vi "main.vi"() -> ()   [LabVIEW 2016]
uses:
  <vilib>/DAQmx/read.llb/DAQmx Read (Analog 2D DBL NChan NSamp).vi
  <vilib>/DAQmx/miscellaneous.llb/DAQmx Fill In Error Info.vi
  QSM-PC (String)/Library/QSM-PC (String).lvlib
  <resource>/objmgr/daqmx.rc
panel:
  out "error out 3":errorcluster caption="错误输出"
  out "控件值:获取全部 2":cluster{"Name":string, "Variant Data":variant}[](array[cluster])
  out "输出簇":T1
  in  "Function":bool
  in  "Oscilloscope":bool
  out "DevName":string
  out "DCVoltage":dbl
  out "ai taskhandle":refnum<k21>
  out "error out read ai":errorcluster caption="error out"
  out "taskArr out create task out":refnum<k21>[](array[refnum])
  out "taskArr out create task in":refnum<k21>[](array[refnum])
  out "isDeviceExist":bool
  out "isNull":bool
  out "taskArr out":refnum<k21>[](array[refnum])
  out "error out 2":errorcluster caption="error out"
  out "error out":errorcluster
  out "msg from wrapper":cluster{"State":string, "Data":variant}
  in  "Creat_Task":bool
  out "AI":dbl[][](array[numeric])
  in  "Search_Drive":bool
  out "控件值:获取全部":cluster{"Name":string, "Variant Data":variant}[](array[cluster])
  out "QSM - Main":refnum<queue>
  out "R":dbl
  in  "调零测量":bool
  in  "start AI":bool
  in  "Stop":bool
  in  "Read R":bool
  in  "event registration refnum":refnum<event-registration>
  in  "user event out":refnum<user-event>
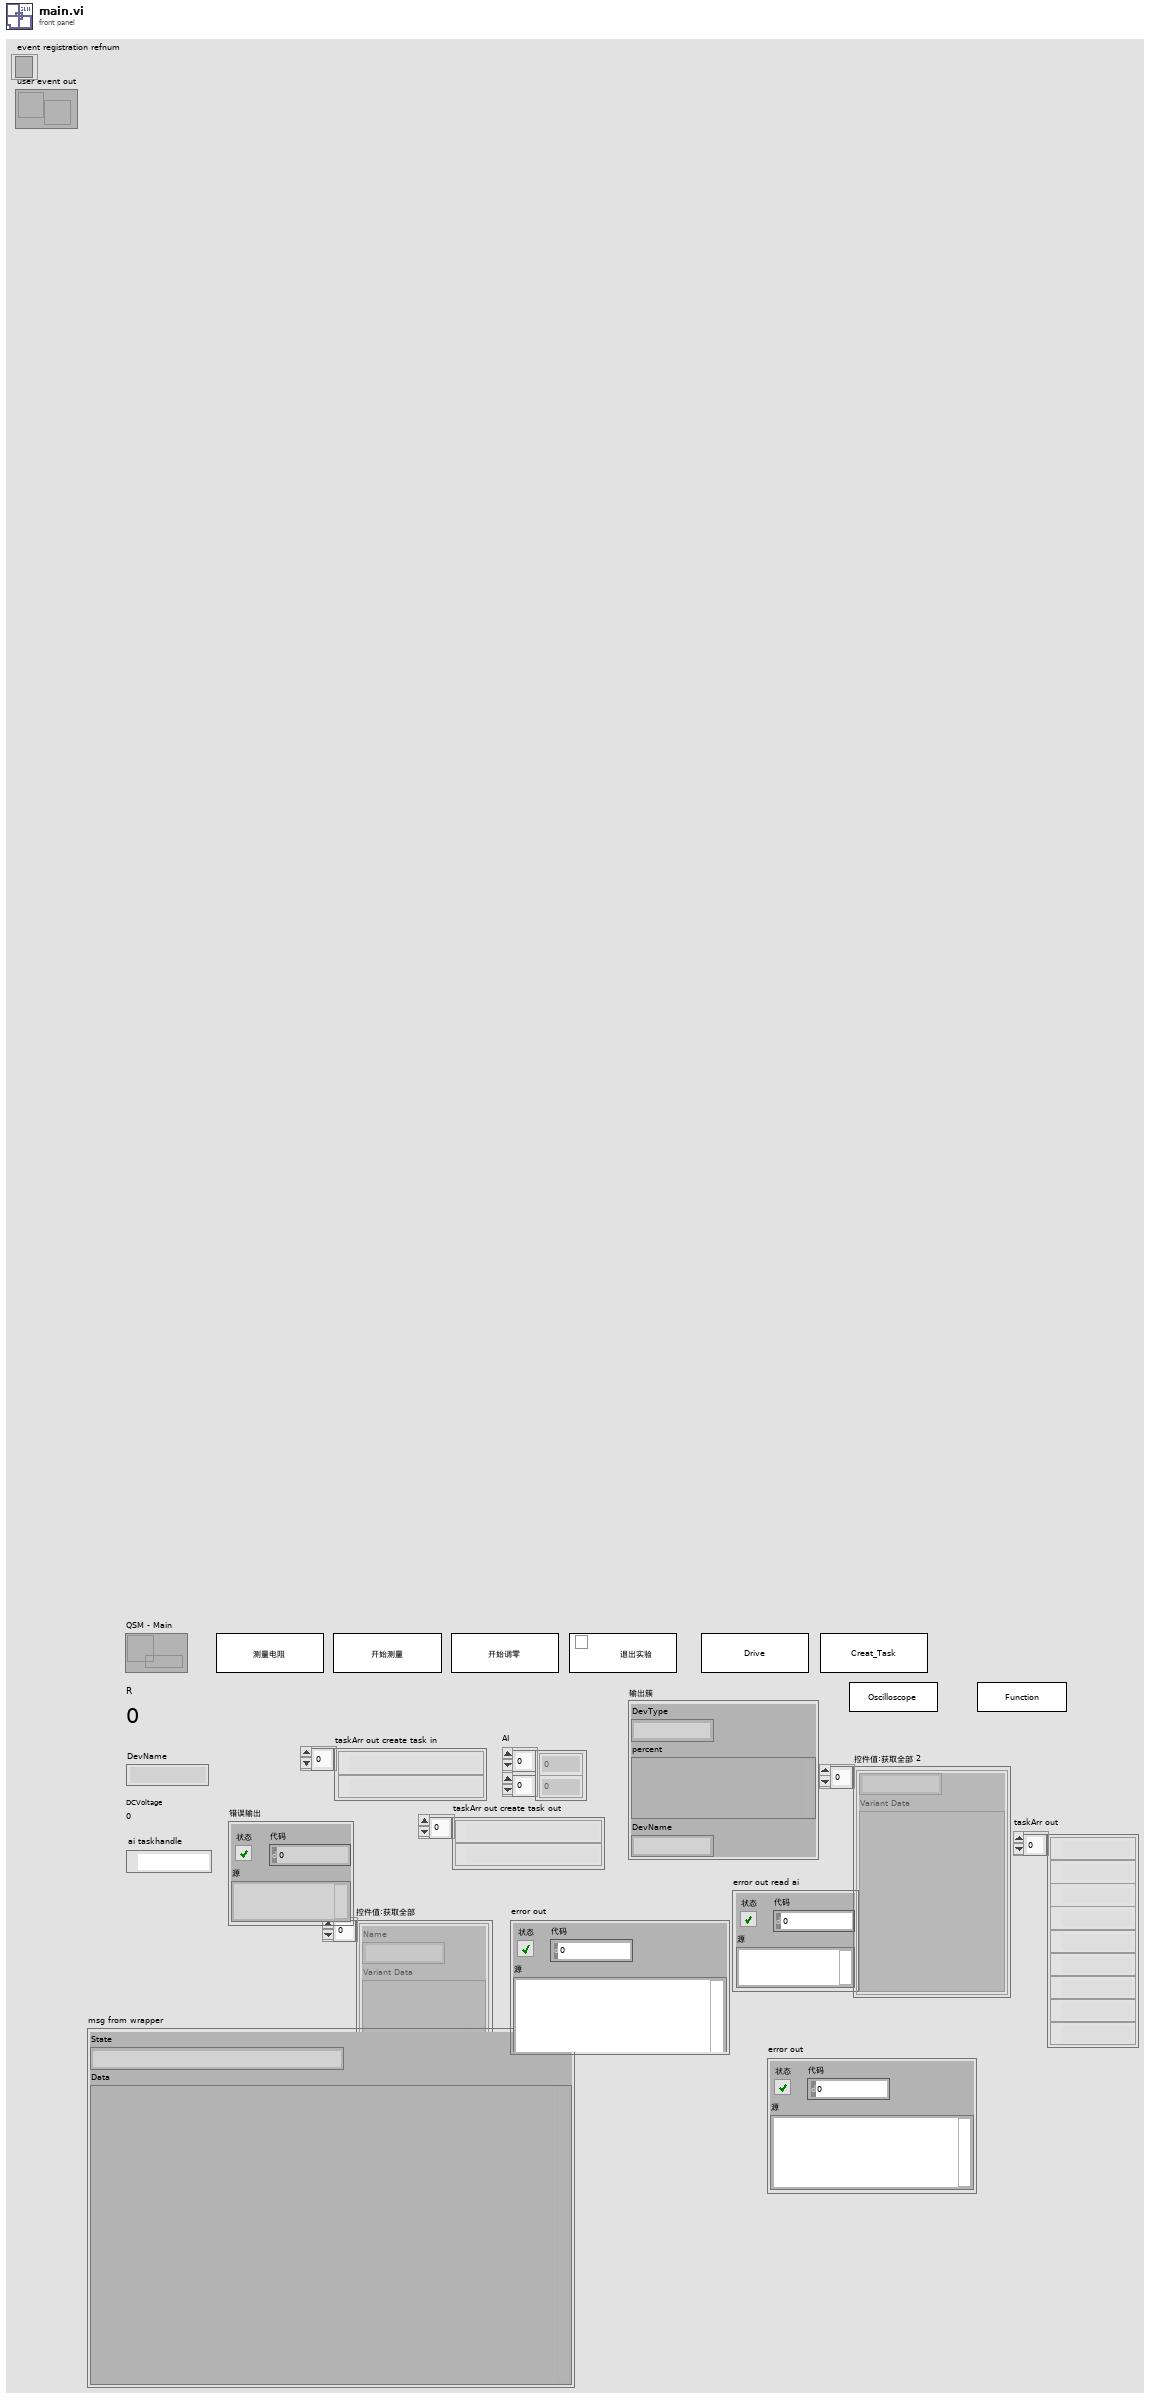
[diagram p1: front panel]
types:
  T1 = cluster{"DevType":string, "percent":variant, "DevName":string}
  T2 = cluster{"Oscilloscope":refnum<queue>, "Function":refnum<queue>}
  T3 = cluster{"DevType":string, "percent":dbl, "DevName":string}
  T4 = cluster{"DevType":string, "DevName":string, "Function":variant}
  T5 = typedef "Configuration.ctl" = cluster{"tasks":T6[]}
  T6 = typedef "TaskConfig.ctl" = cluster{"type":string, "channels":T7[], "sampleclock":T8}
  T7 = typedef "ChanConfig.ctl" = cluster{"physicalchanname":string, "max":dbl, "min":dbl}
  T8 = typedef "ClockConfig.ctl" = cluster{"rate":dbl, "samplesperchannel":i32}
  T9 = cluster{"Config":T5, "DevName":string, "DevType":string}
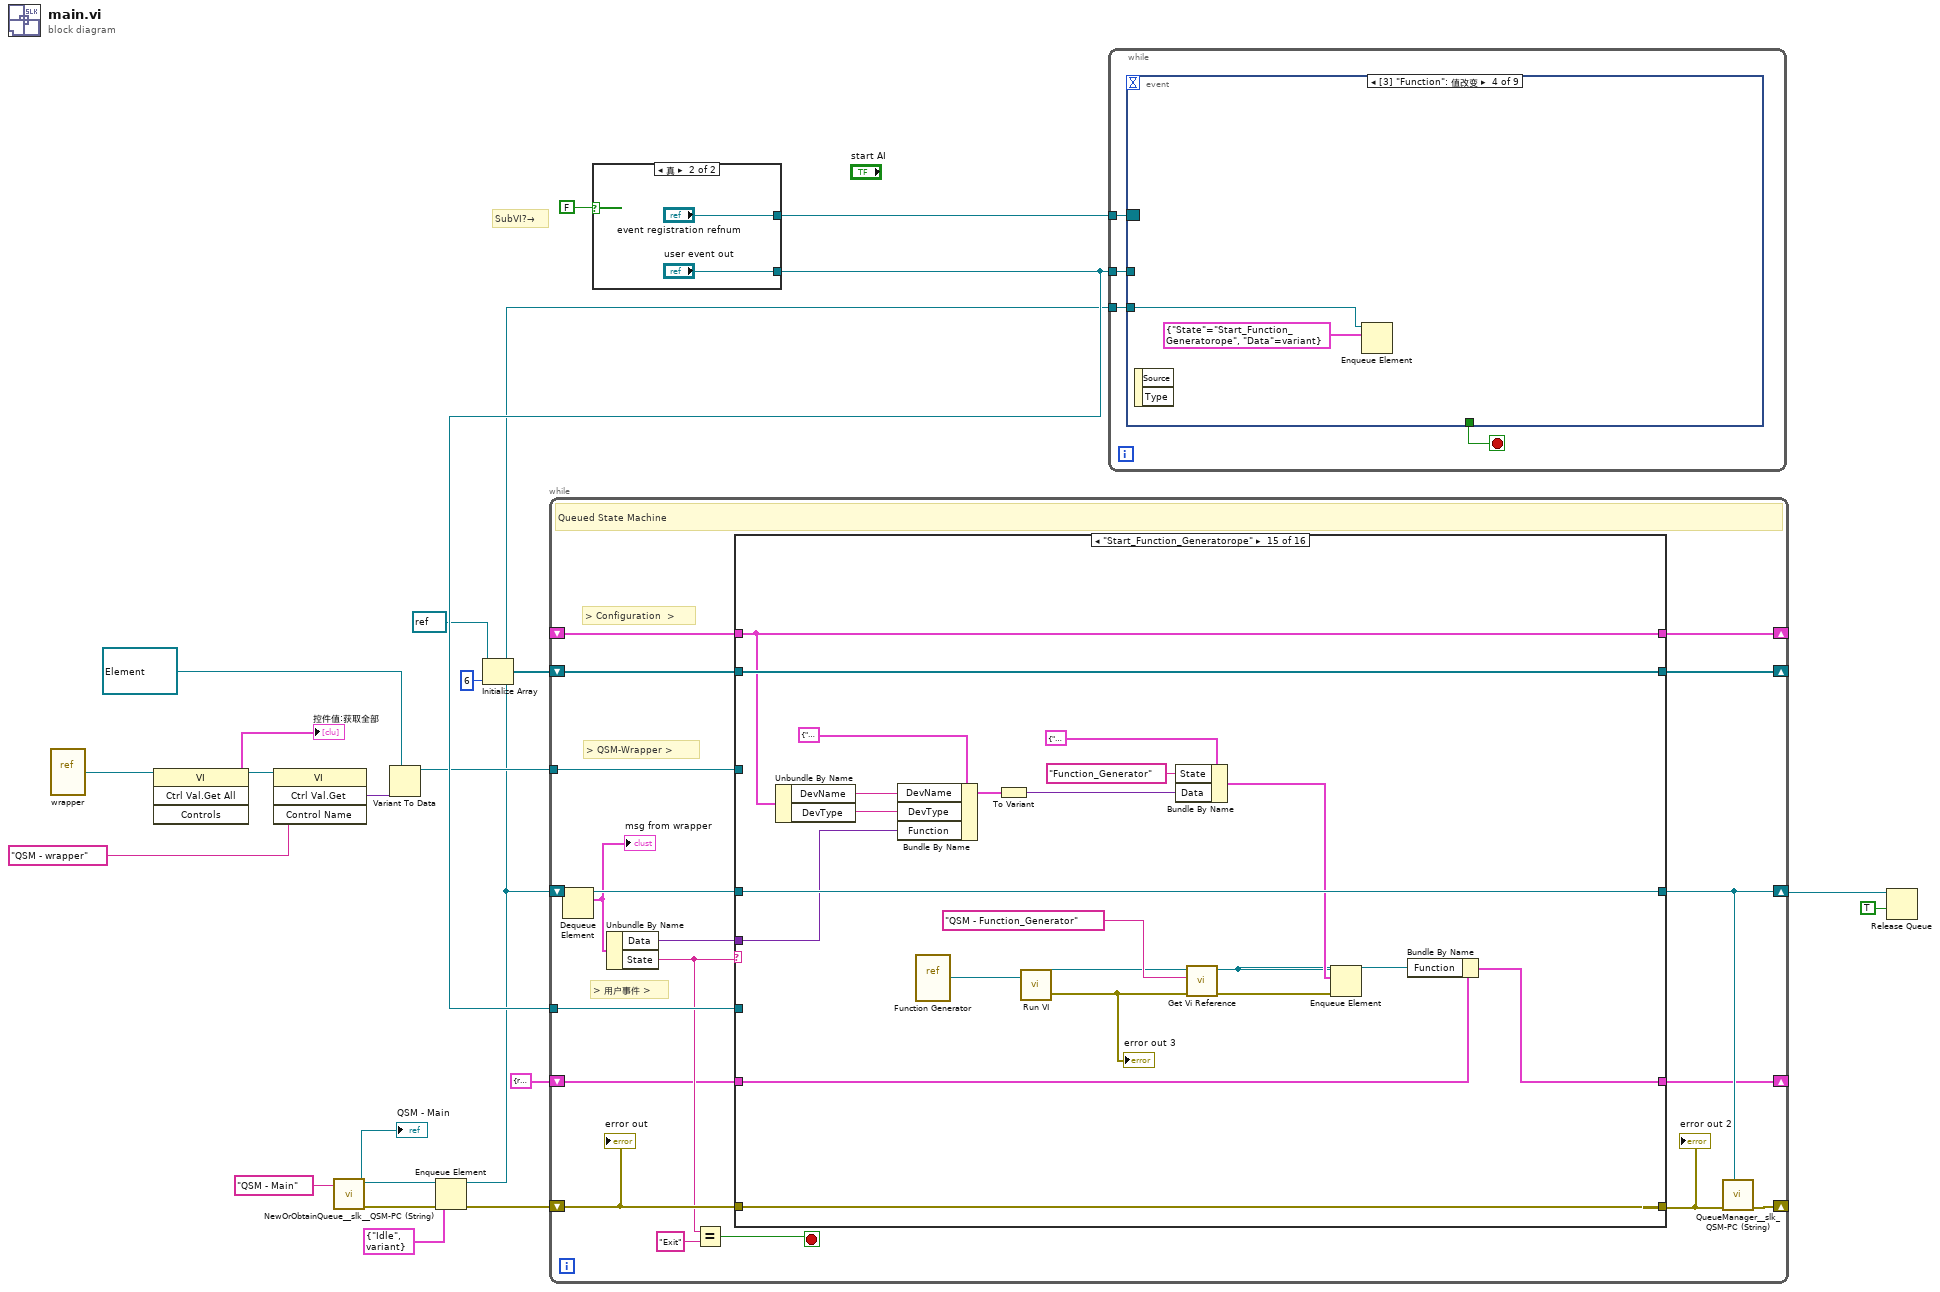
[diagram p0: block diagram]
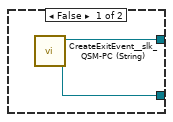
[diagram p2: hidden frame]
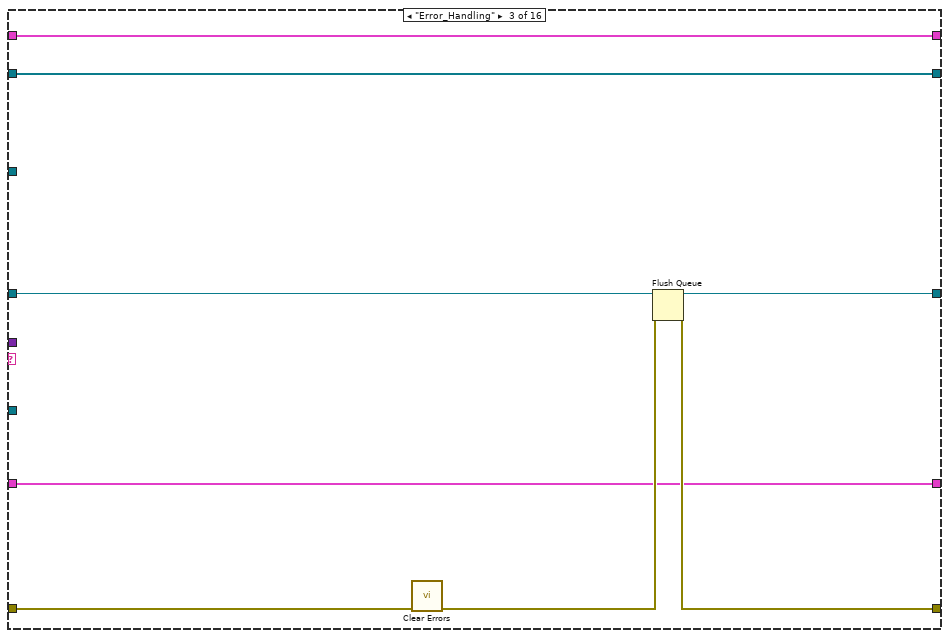
[diagram p5: hidden frame]
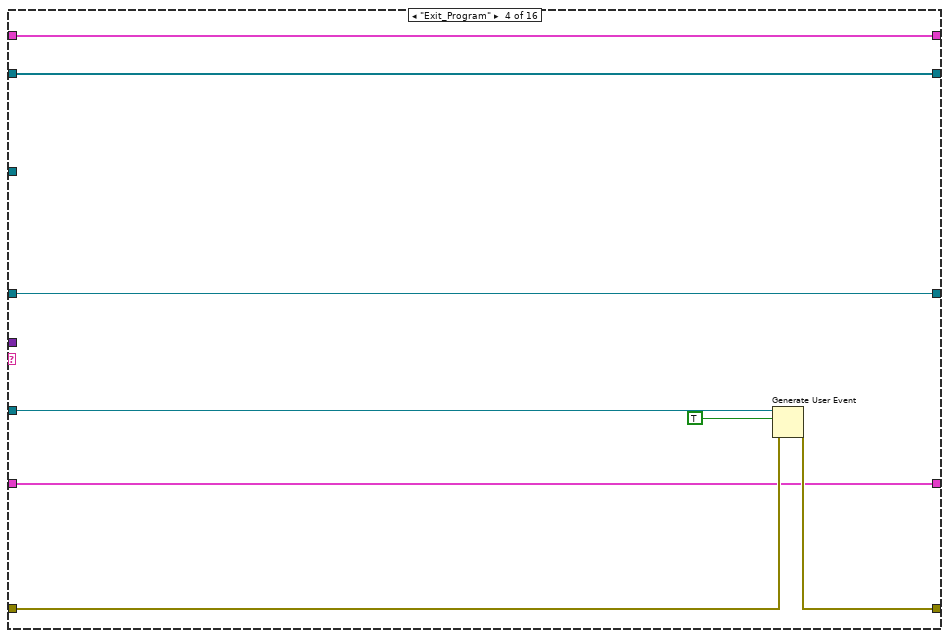
[diagram p6: hidden frame]
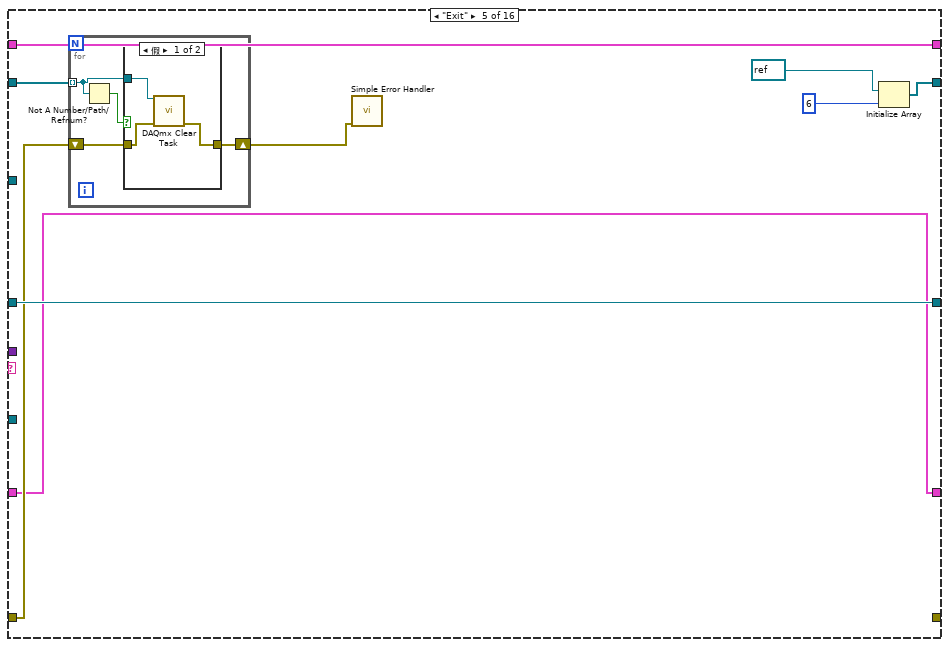
[diagram p7: hidden frame]
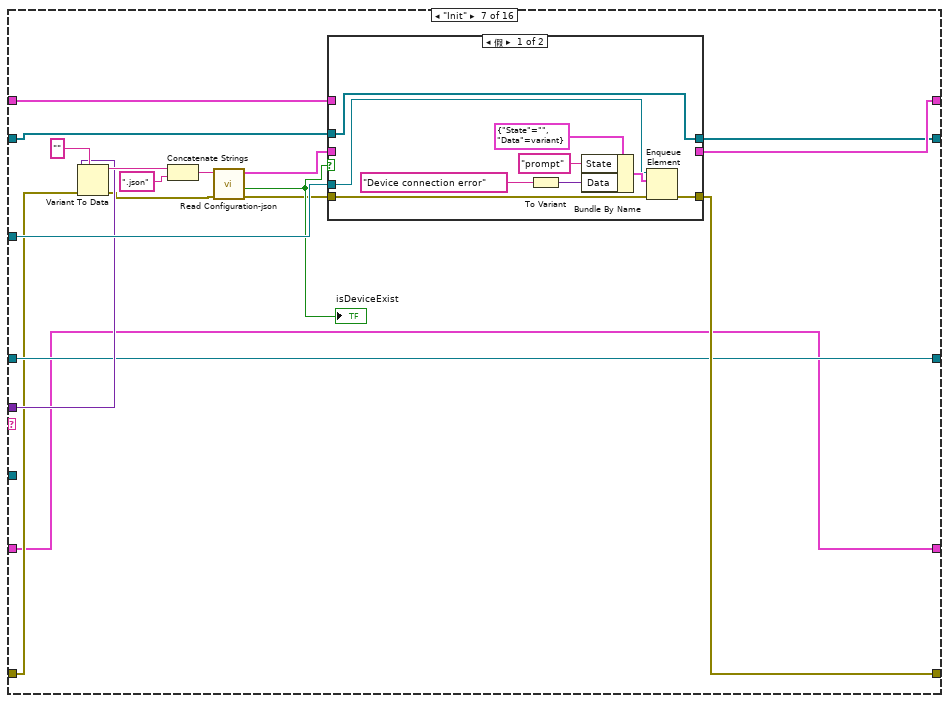
[diagram p10: hidden frame]
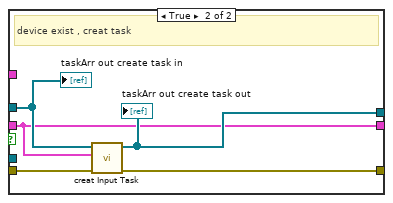
[diagram p11: hidden frame]
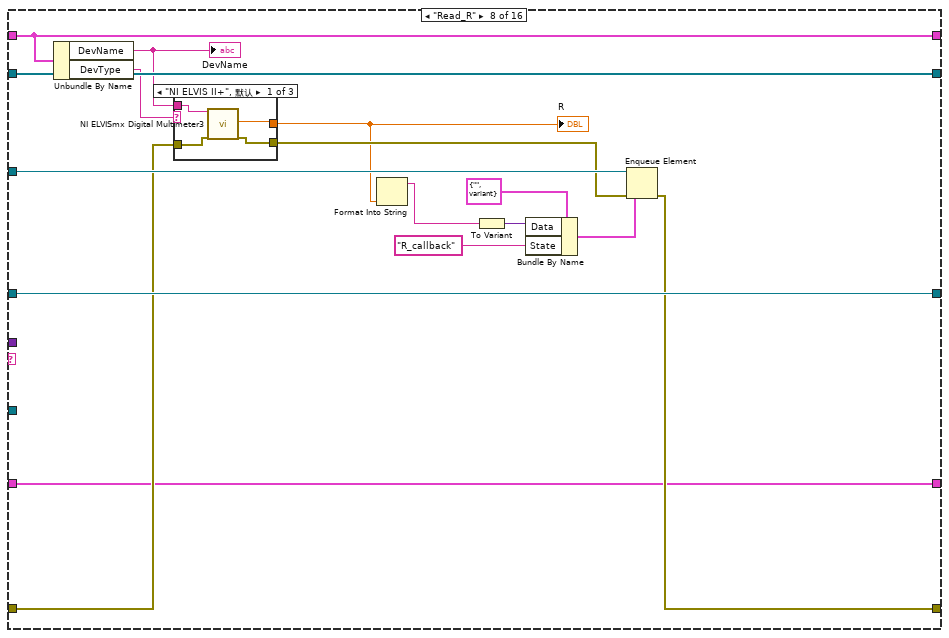
[diagram p12: hidden frame]
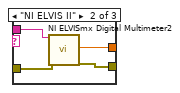
[diagram p13: hidden frame]
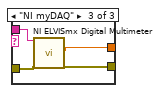
[diagram p14: hidden frame]
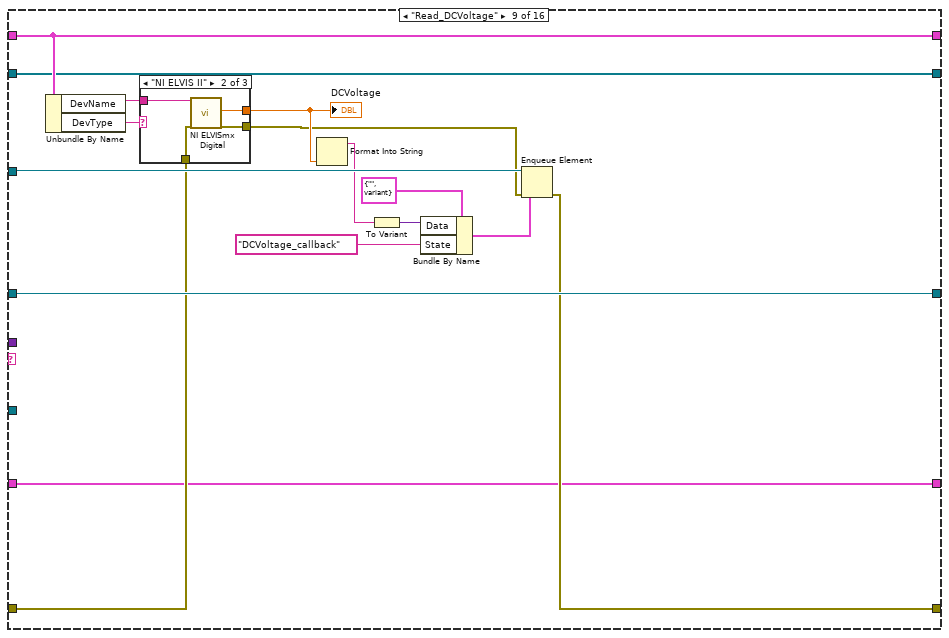
[diagram p15: hidden frame]
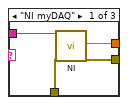
[diagram p16: hidden frame]
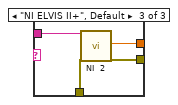
[diagram p17: hidden frame]
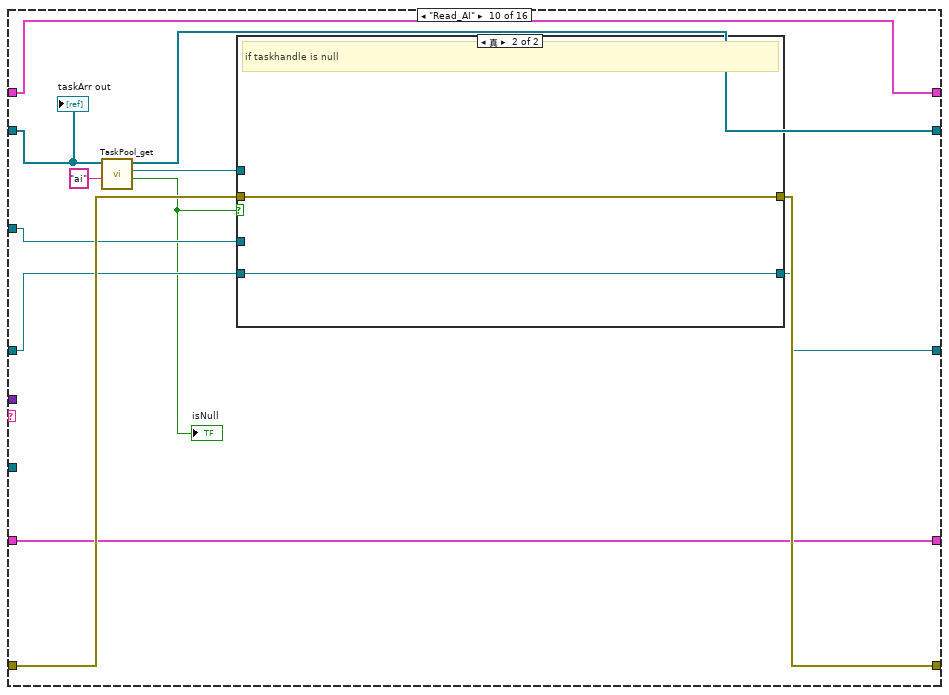
[diagram p18: hidden frame]
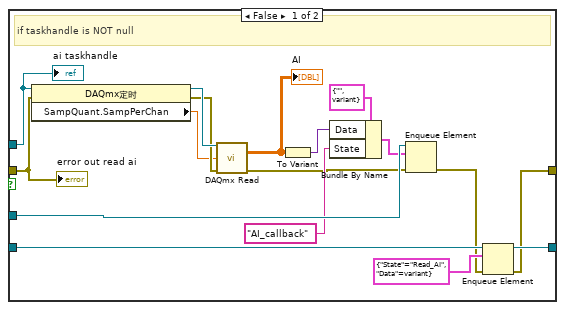
[diagram p19: hidden frame]
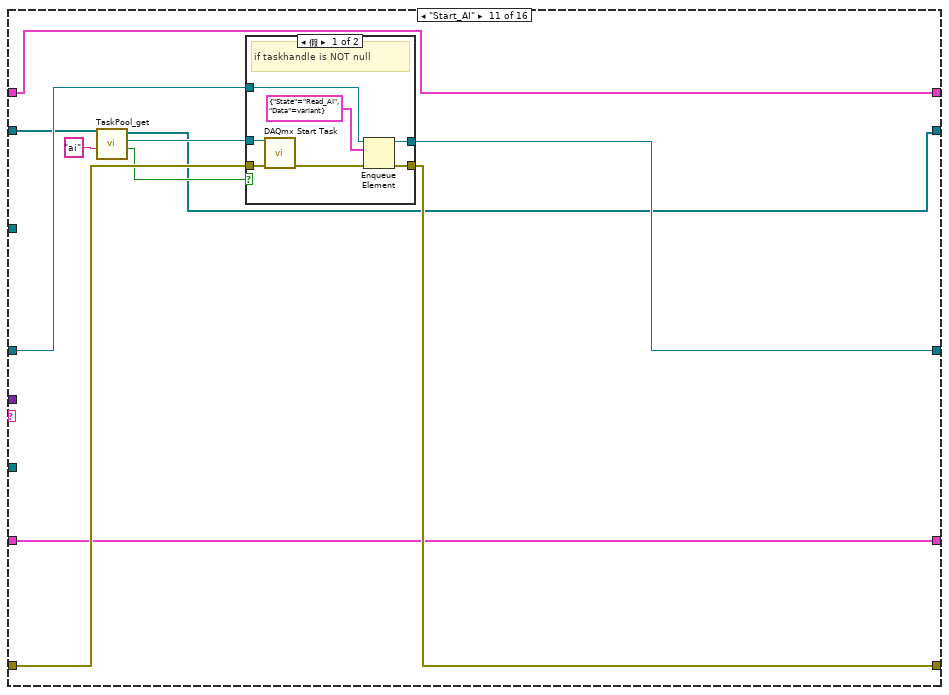
[diagram p20: hidden frame]
diagram:
  # "SubVI?→"
  n1 = vi-ref "wrapper.vi"() -> (w14:refnum<vi>)
  n2 = invoke class="VI" method="Ctrl Val.Get All"(reference=w14) -> (reference out=w15:refnum<vi>, "Get All Control Values Variant"=→"控件值:获取全部":cluster{"Name":string, "Variant Data":variant}[])  [unwired: 3 in, 2 out]
  n3 = invoke class="VI" method="Ctrl Val.Get"(reference=w15, "Control Name"="QSM - wrapper" ("控件名")) -> ("Get Control Value Variant"=w16:variant)  [unwired: 2 in, 3 out]
  n4 = call "NewOrObtainQueue__slk__QSM-PC (String).vi"("queue name in"="QSM - Main" ("控件名")) -> ("error out"=w9:errorcluster, "queue out"=w11:refnum<queue>)  [unwired: 2 in, 7 out]
  "QSM - Main" <- w11
  n5 = Variant To Data(type=refnum<queue> refnum ("队列输出"), Variant=w16) -> (data=w13:refnum<queue>)  [unwired: 1 in, 1 out]
  n6 = Enqueue Element(queue=w11, element=cluster{"State":string, "Data":variant} {"State"="Idle", "Data"=variant} ("元素"), error in (no error)=w9) -> (queue out=w10:refnum<queue>, error out=w8:errorcluster)  [unwired: 2 out]
  n7 = Initialize Array(refnum<k21> refnum ("task out"), 6 ("维数大小")) -> (w3:refnum<k21>[])
  n8 = case shown="真" FALSE {
    tunnel: [w24 "event registration refnum"] -> w22
    tunnel: [w23 "user event out"] -> w18
    frame False {
      n9 = call "CreateExitEvent__slk_QSM-PC (String).vi"() -> ("user event out"=w23:refnum<user-event>, "event registration refnum out"=w24:refnum<event-registration>)  [unwired: 10 out]
    }
    frame True {
    }
  }
  n10 = while {
    shift-right: [w40] -> _
    shift-left: w8 -> [w39]
    shift-right: [w37] -> w21
    shift-left: w10 -> [w45]
    tunnel: w18 -> [w38]
    tunnel: w13 -> [w35]
    shift-right: [w33] -> _
    shift-left: _ -> [w34]
    shift-right: [w30] -> _
    shift-left: w3 -> [w31]
    shift-right: [w27] -> _
    shift-left: T2 {"Oscilloscope"=refnum, "Function"=refnum} ("Sub VI Reference") -> [w28]
    stop <- w36 stop-if-true
    # "> Configuration  >"
    # "> 用户事件 >"
    # "> QSM-Wrapper >"
    # "Queued State Machine"
    n11 = Dequeue Element(queue=w45) -> (queue out=w41:refnum<queue>, element=w29:cluster{"State":string, "Data":variant})  [unwired: 1 in, 3 out]
    "msg from wrapper" <- w29
    n12 = Unbundle By Name(w29) -> ("Data"=w44:variant, "State"=w32:string)
    n13 = Equal?(x=w32, y="Exit") -> (x = y?=w36:bool)
    n14 = case shown="\"Start_Function_Generatorope\"" w32 {
      tunnel: w44 -> [_ _ _ _ _ _ w103 _ _ _ _ _ w253 _ w287 _]
      tunnel: w39 -> [w48 w55 w59 w67 w77 w93 w96 w129 w157 w193 w220 w241 w269 w278 w299 w308]
      tunnel: [w48 w55 w61 w68 _ w93 w104 w133 w161 w192 w221 w240 w269 w278 w299 w308] -> w43
      tunnel: w35 -> [_ _ _ _ _ _ w107 w140 w163 w191 _ _ _ _ _ _]
      tunnel: w41 -> [w50 w54 w63 w71 w80 w92 w98 w141 w162 w189 w223 w242 w259 w275 w297 w307]
      tunnel: [w50 w54 w60 w71 w80 w92 w98 w141 w162 w190 w222 w242 w259 w275 w297 w307] -> w37
      tunnel: w38 -> [_ _ _ w69 _ _ _ _ _ _ _ _ _ _ _ _]
      tunnel: w34 -> [w49 w53 w58 w66 w79 w91 w99 w135 w169 w184 w215 w239 w251 w277 w290 w306]
      tunnel: [w49 w53 w58 w66 w79 w91 w100 w135 w169 w184 w215 w239 w251 w277 w290 w306] -> w33
      tunnel: w31 -> [w47 w52 w57 w65 w78 w90 w102 w134 w168 w188 w218 w237 w268 w276 w298 w305]
      tunnel: [w47 w52 w57 w65 w73 w90 w97 w134 w168 w183 w214 w235 w268 w276 w298 w305] -> w30
      tunnel: w28 -> [w46 w51 w56 w64 w72 w89 w94 w126 w154 w182 w213 w233 w265 w270 w296 w304]
      tunnel: [w46 w51 w56 w64 w72 w89 w94 w126 w154 w182 w213 w233 w264 w270 w295 w304] -> w27
      frame "-----internal-----" {
      }
      frame "Idle", Default {
      }
      frame "Error_Handling" {
        n15 = call <vilib>:"Clear Errors.vi"("error in (no error)"=w59) -> ("error out"=w62:errorcluster)  [unwired: 5 in, 1 out]
        n16 = Flush Queue(queue=w63, error in (no error)=w62) -> (queue out=w60:refnum<queue>, error out=w61:errorcluster)  [unwired: 1 out]
      }
      frame "Exit_Program" {
        n17 = Generate User Event(user event=w69, event data cluster=TRUE ("event data"), error in=w67) -> (error out=w68:errorcluster)  [unwired: 1 in, 1 out]
      }
      frame "Exit" {
        n18 = for {
          tunnel: w78 -> [w83] mode=indexing
          shift-right: [w81] -> w76
          shift-left: w77 -> [w82]
          n19 = Not A Number/Path/Refnum?(number/path/refnum=w83) -> (NaN/Path/Refnum?=w84:bool)
          n20 = case shown="假" w84 {
            tunnel: [w87 w88] -> w81
            tunnel: w83 -> [w86 _]
            tunnel: w82 -> [w85 w88]
            frame False {
              n21 = call <vilib>:"DAQmx Clear Task.vi"("task in"=w86, "error in"=w85) -> ("error out"=w87:errorcluster)  [unwired: 13 in]
            }
            frame True {
            }
          }
        }
        n22 = call <vilib>:"Simple Error Handler.vi"("error in (no error)"=w76) -> ()  [unwired: 4 in, 5 out]
        n23 = Initialize Array(refnum<k21> refnum ("task out"), 6 ("维数大小")) -> (w73:refnum<k21>[])
      }
      frame "-----public-----" {
      }
      frame "Init" {
        n24 = Variant To Data(error in=w96, type="", Variant=w103) -> (data=w109:string, error out=w95:errorcluster)
        n25 = Concatenate Strings(w109, ".json" ("字符串")) -> (w108:string)
        n26 = call "Read Configuration-json.vi"("error in (no error)"=w95, "Filename"=w108) -> ("error out"=w105:errorcluster, "isDeviceExist"=w106:bool, "Configuration"=w101:T9)  [unwired: 7 in]
        "isDeviceExist" <- w106
        n27 = case shown="假" w106 {
          tunnel: w107 -> [w115 _]
          tunnel: w105 -> [w113 w125]
          tunnel: [w112 w124] -> w104
          tunnel: [w114 w123] -> w97
          tunnel: w102 -> [w114 w122]
          tunnel: w101 -> [_ w121]
          tunnel: [_ w121] -> w100
          tunnel: w99 -> [_ _]
          frame False {
            n28 = To Variant(anything="Device connection error" ("State")) -> (Variant=w117:variant)
            n29 = Bundle By Name(cluster=cluster{"State":string, "Data":variant} {"State"="", "Data"=variant} ("元素"), "State"="prompt", "Data"=w117) -> (w120:cluster{"State":string, "Data":variant})
            n30 = Enqueue Element(queue=w115, element=w120, error in (no error)=w113) -> (error out=w112:errorcluster)  [unwired: 3 out]
          }
          frame True {
            # "device exist , creat task"
            n31 = call "creat Input Task.vi"("error in"=w125, "Configuration"=w121, "taskArr in"=w122) -> ("error out"=w124:errorcluster, "taskArr out"=w123:refnum<k21>[])  [unwired: 7 in]
            "taskArr out create task out" <- w123
            "taskArr out create task in" <- w122
          }
        }
      }
      frame "Read_R" {
        n32 = Unbundle By Name(w135) -> ("DevName"=w130:string, "DevType"=w131:string)
        "DevName" <- w130
        n33 = case shown="\"NI ELVIS II+\", 默认" w131 {
          tunnel: w130 -> [w145 w147 w153]
          tunnel: w129 -> [w144 w148 w152]
          tunnel: [w142 w149 w151] -> w128
          tunnel: [w143 w146 w150] -> w127
          frame "NI ELVIS II+", Default {
            n34 = call "NI ELVISmx Digital Multimeter3"("Device Name"=w145, "error in"=w144) -> ("Measurement"=w143:dbl, "error out"=w142:errorcluster)  [unwired: 15 in, 1 out]
          }
          frame "NI ELVIS II" {
            n35 = call "NI ELVISmx Digital Multimeter2"("Device Name"=w147, "error in"=w148) -> ("Measurement"=w146:dbl, "error out"=w149:errorcluster)  [unwired: 15 in, 1 out]
          }
          frame "NI myDAQ" {
            n36 = call "NI ELVISmx Digital Multimeter"("Device Name"=w153, "error in"=w152) -> ("Measurement"=w150:dbl, "error out"=w151:errorcluster)  [unwired: 15 in, 1 out]
          }
        }
        "R" <- w127
        n37 = Format Into String(w127) -> (resulting string=w132:string)  [unwired: 3 in, 1 out]
        n38 = To Variant(anything=w132) -> (Variant=w137:variant)
        n39 = Bundle By Name(cluster=cluster{"State":string, "Data":variant} {"State"="", "Data"=variant} ("元素"), "Data"=w137, "State"="R_callback") -> (w138:cluster{"State":string, "Data":variant})
        n40 = Enqueue Element(queue=w140, element=w138, error in (no error)=w128) -> (error out=w133:errorcluster)  [unwired: 3 out]
      }
      frame "Read_DCVoltage" {
        n41 = Unbundle By Name(w169) -> ("DevName"=w158:string, "DevType"=w159:string)
        n42 = case shown="\"NI ELVIS II\"" w159 {
          tunnel: w158 -> [w173 w177 w178]
          tunnel: w157 -> [w172 w176 w179]
          tunnel: [w171 w175 w180] -> w155
          tunnel: [w170 w174 w181] -> w156
          frame "NI myDAQ" {
            n43 = call "NI"("Device Name"=w173, "error in"=w172) -> ("Measurement"=w170:dbl, "error out"=w171:errorcluster)  [unwired: 15 in, 1 out]
          }
          frame "NI ELVIS II" {
            n44 = call "NI ELVISmx Digital"("Device Name"=w177, "error in"=w176) -> ("Measurement"=w174:dbl, "error out"=w175:errorcluster)  [unwired: 15 in, 1 out]
          }
          frame "NI ELVIS II+", Default {
            n45 = call "NI  2"("Device Name"=w178, "error in"=w179) -> ("Measurement"=w181:dbl, "error out"=w180:errorcluster)  [unwired: 15 in, 1 out]
          }
        }
        "DCVoltage" <- w156
        n46 = Format Into String(w156) -> (resulting string=w160:string)  [unwired: 3 in, 1 out]
        n47 = To Variant(anything=w160) -> (Variant=w165:variant)
        n48 = Bundle By Name(cluster=cluster{"State":string, "Data":variant} {"State"="", "Data"=variant} ("元素"), "Data"=w165, "State"="DCVoltage_callback") -> (w166:cluster{"State":string, "Data":variant})
        n49 = Enqueue Element(queue=w163, element=w166, error in (no error)=w155) -> (error out=w161:errorcluster)  [unwired: 3 out]
      }
      frame "Read_AI" {
        n50 = call "TaskPool_get.vi"("taskType"="ai", "taskArr in"=w188) -> ("isNull"=w186:bool, "taskhandle"=w185:refnum<k21>, "taskArr out"=w183:refnum<k21>[])  [unwired: 6 in]
        "isNull" <- w186
        n51 = case shown="真" w186 {
          tunnel: w193 -> [w199 w212]
          tunnel: [w194 w212] -> w192
          tunnel: w191 -> [w210 _]
          tunnel: [w208 w211] -> w190
          tunnel: w189 -> [w207 w211]
          tunnel: w185 -> [w201 _]
          frame False {
            # "if taskhandle is NOT null"
            n52 = property class="DAQmx定时"(reference=w201, error in=w199) -> (reference out=w200:refnum<k21>, error out=w198:errorcluster, "SampQuant.SampPerChan"=w197:dbl)
            n53 = call-poly <vilib>:"DAQmx Read.vi"("task/channels in"=w200, "number of samples per channel"=w197, "error in"=w198) -> ("data"=w209:dbl[][], "error out"=w196:errorcluster)  [unwired: 10 in, 1 out]
            "AI" <- w209
            n54 = To Variant(anything=w209) -> (Variant=w203:variant)
            n55 = Bundle By Name(cluster=cluster{"State":string, "Data":variant} {"State"="", "Data"=variant} ("元素"), "Data"=w203, "State"="AI_callback") -> (w205:cluster{"State":string, "Data":variant})
            n56 = Enqueue Element(queue=w210, element=w205, error in (no error)=w196) -> (error out=w195:errorcluster)  [unwired: 3 out]
            n57 = Enqueue Element(queue=w207, element=cluster{"State":string, "Data":variant} {"State"="Read_AI", "Data"=variant} ("元素"), error in (no error)=w195) -> (queue out=w208:refnum<queue>, error out=w194:errorcluster)  [unwired: 2 out]
            "error out read ai" <- w199
            "ai taskhandle" <- w201
          }
          frame True {
            # "if taskhandle is null"
          }
        }
        "taskArr out" <- w188
      }
      frame "Start_AI" {
        n58 = call "TaskPool_get.vi"("taskType"="ai", "taskArr in"=w218) -> ("isNull"=w217:bool, "taskhandle"=w216:refnum<k21>, "taskArr out"=w214:refnum<k21>[])  [unwired: 6 in]
        n59 = case shown="假" w217 {
          tunnel: w223 -> [w230 w232]
          tunnel: [w228 w232] -> w222
          tunnel: [w227 w231] -> w221
          tunnel: w220 -> [w226 w231]
          tunnel: w216 -> [w224 _]
          frame False {
            # "if taskhandle is NOT null"
            n60 = call <vilib>:"DAQmx Start Task.vi"("task/channels in"=w224, "error in"=w226) -> ("error out"=w225:errorcluster)  [unwired: 12 in, 1 out]
            n61 = Enqueue Element(queue=w230, element=cluster{"State":string, "Data":variant} {"State"="Read_AI", "Data"=variant} ("Element"), error in (no error)=w225) -> (queue out=w228:refnum<queue>, error out=w227:errorcluster)  [unwired: 2 out]
          }
          frame True {
            # "if taskhandle is null"
          }
        }
      }
      frame "Stop_AI" {
        n62 = call "TaskPool_get.vi"("taskType"="ai", "taskArr in"=w237) -> ("isNull"=w236:bool, "taskhandle"=w234:refnum<k21>, "taskArr out"=w235:refnum<k21>[])  [unwired: 6 in]
        n63 = case shown="假" w236 {
          tunnel: w241 -> [w245 w246]
          tunnel: [w244 w246] -> w240
          tunnel: w234 -> [w243 _]
          frame False {
            n64 = call <vilib>:"DAQmx Stop Task.vi"("task/channels in"=w243, "error in"=w245) -> ("error out"=w244:errorcluster)  [unwired: 12 in, 1 out]
          }
          frame True {
          }
        }
      }
      frame "Start_Oscilloscope" {
        n65 = Unbundle By Name(w251) -> ("DevType"=w257:string, "DevName"=w256:string)
        n66 = Variant To Data(type=0.0 ("percent"), Variant=w253) -> (data=w252:dbl)  [unwired: 1 in, 1 out]
        n67 = Bundle By Name(cluster=T3 {"DevType"="", "percent"=0.0, "DevName"=""}, "DevType"=w257, "DevName"=w256, "percent"=w252) -> (w255:T3)
        "输出簇" <- w255
        n68 = vi-ref "Oscilloscope.vi"() -> (w248:refnum<vi>)
        n69 = call "Run VI.vi"("VI Reference in"=w248) -> ("error out"=w249:errorcluster, "VI Reference out"=w247:refnum<vi>)  [unwired: 1 in]
        n70 = Bundle By Name(cluster=cluster{"State":string, "Data":variant} {"State"="", "Data"=variant} ("元素"), "State"=" Read_Oscilloscope", "Data"=w255) -> (w261:cluster{"State":string, "Data":variant})
        n71 = call "Get Vi Reference.vi"("error in (no error)"=w249, "Control name"="QSM - Oscilloscope", "Vi Reference in"=w247) -> ("error out"=w266:errorcluster, "控件值:获取全部"=→"控件值:获取全部 2":cluster{"Name":string, "Variant Data":variant}[], "队列输出"=w263:refnum<queue>)  [unwired: 5 in]
        n72 = Bundle By Name(cluster=w265, "Oscilloscope"=w263) -> (w264:T2)
        n73 = Enqueue Element(queue=w263, element=w261, error in (no error)=w266) -> ()  [unwired: 1 in, 3 out]
      }
      frame "Stop_Oscilloscope" {
        n74 = Unbundle By Name(w270) -> ("Oscilloscope"=w274:refnum<queue>)
        n75 = Bundle By Name(cluster=cluster{"State":string, "Data":variant} {"State"="", "Data"=variant} ("元素"), "State"="Exit") -> (w272:cluster{"State":string, "Data":variant})
        n76 = Enqueue Element(queue=w274, element=w272) -> ()  [unwired: 2 in, 3 out]
      }
      frame "Start_Function_Generatorope" {
        n77 = Unbundle By Name(w290) -> ("DevName"=w288:string, "DevType"=w289:string)
        n78 = Bundle By Name(cluster=T4 {"DevType"="", "DevName"="", "Function"=variant}, "DevName"=w288, "DevType"=w289, "Function"=w287) -> (w285:T4)
        n79 = vi-ref "Function Generator.vi"() -> (w283:refnum<vi>)
        n80 = To Variant(anything=w285) -> (Variant=w286:variant)
        n81 = call "Run VI.vi"("VI Reference in"=w283) -> ("error out"=w279:errorcluster, "VI Reference out"=w282:refnum<vi>)  [unwired: 1 in]
        "error out 3" <- w279
        n82 = Bundle By Name(cluster=cluster{"State":string, "Data":variant} {"State"="", "Data"=variant} ("元素"), "State"="Function_Generator", "Data"=w286) -> (w293:cluster{"State":string, "Data":variant})
        n83 = call "Get Vi Reference.vi"("error in (no error)"=w279, "Control name"="QSM - Function_Generator", "Vi Reference in"=w282) -> ("error out"=w280:errorcluster, "队列输出"=w281:refnum<queue>)  [unwired: 5 in, 1 out]
        n84 = Enqueue Element(queue=w281, element=w293, error in (no error)=w280) -> ()  [unwired: 1 in, 3 out]
        n85 = Bundle By Name(cluster=w296, "Function"=w281) -> (w295:T2)
      }
      frame "Stop_Function_Generator" {
        n86 = Unbundle By Name(w304) -> ("Function"=w303:refnum<queue>)
        n87 = Bundle By Name(cluster=cluster{"State":string, "Data":variant} {"State"="", "Data"=variant} ("元素"), "State"="Exit") -> (w301:cluster{"State":string, "Data":variant})
        n88 = Enqueue Element(queue=w303, element=w301) -> ()  [unwired: 2 in, 3 out]
      }
    }
    "error out 2" <- w43
    n89 = call "QueueManager__slk_QSM-PC (String).vi"("queue in"=w37, "error in (no error)"=w43) -> ("error out"=w40:errorcluster)  [unwired: 2 in, 7 out]
    "error out" <- w39
  }
  n90 = while {
    tunnel: w22 -> [w312]
    tunnel: w18 -> [w311]
    tunnel: w10 -> [w310]
    stop <- w309 stop-if-true
    n91 = event shown="[3] \"Function\": 值改变" {
      selector: w312 -> [_ _ _ _ _ _ _ _ _]
      dyn-events: _ -> [_ _ _ _ _ _ _ _ _]
      timeout: _ -> [_ _ _ _ _ _ _ _ _]
      tunnel: w311 -> [w316 _ _ _ _ _ _ _ _]
      tunnel: w310 -> [w313 w319 w320 w322 w325 w332 w339 w341 w343]
      tunnel: [w315 w318 _ _ FALSE ("Exit") FALSE ("Exit") FALSE ("Exit") _ _] -> w309
      event "Stop": Value Change {
        w315 = TRUE
        n92 = event-data() -> ()  [unwired: 2 out]
        n93 = Enqueue Element(queue=w313, element=cluster{"State":string, "Data":variant} {"State"="Exit", "Data"=variant} ("Element")) -> ()  [unwired: 1 in, 4 out]
        n94 = Generate User Event(user event=w316, event data cluster=w315) -> ()  [unwired: 2 in, 2 out]
      }
      event User Event {
        # "Event-Handling Loop"
        n95 = event-data() -> ("Exit"=w318:bool)  [unwired: 1 out]
        n96 = Enqueue Element(queue=w319, element=cluster{"State":string, "Data":variant} {"State"="Exit", "Data"=variant} ("Element")) -> ()  [unwired: 1 in, 4 out]
      }
      event "Oscilloscope": Value Change {
        n97 = event-data() -> ()  [unwired: 3 out]
        n98 = Enqueue Element(queue=w320, element=cluster{"State":string, "Data":variant} {"State"="Start_Oscilloscope", "Data"=variant} ("Element")) -> ()  [unwired: 1 in, 4 out]
      }
      event "Function": Value Change {
        n99 = event-data() -> ()  [unwired: 3 out]
        n100 = Enqueue Element(queue=w322, element=cluster{"State":string, "Data":variant} {"State"="Start_Function_Generatorope", "Data"=variant} ("Element")) -> ()  [unwired: 1 in, 4 out]
      }
      event "start AI": Value Change {
        n101 = event-data() -> ("NewVal"=w326:bool)  [unwired: 2 out]
        n102 = case shown="真" w326 {
          tunnel: w325 -> [w327 w330]
          frame False {
            n103 = Enqueue Element(queue=w327, element=cluster{"State":string, "Data":variant} {"State"="Stop_AI", "Data"=variant} ("Element")) -> ()  [unwired: 2 in, 3 out]
          }
          frame True {
            n104 = Enqueue Element(queue=w330, element=cluster{"State":string, "Data":variant} {"State"="Start_AI", "Data"=variant} ("Element")) -> ()  [unwired: 2 in, 3 out]
          }
        }
      }
      event "调零测量": Value Change {
        n105 = event-data() -> ("NewVal"=w334:bool)  [unwired: 1 out]
        n106 = case shown="真" w334 {
          tunnel: [cluster{"State":string, "Data":variant} {"State"="Stop_AI", "Data"=variant} ("Element") cluster{"State":string, "Data":variant} {"State"="Start_AI", "Data"=variant} ("Element")] -> w333
          frame False {
          }
          frame True {
          }
        }
        n107 = Flush Queue(queue=w332) -> (queue out=w331:refnum<queue>)  [unwired: 1 in, 2 out]
        n108 = Enqueue Element(queue=w331, element=w333) -> ()  [unwired: 1 in, 4 out]
      }
      event "Search_Drive": Value Change {
        n109 = event-data() -> ()  [unwired: 2 out]
        n110 = Enqueue Element(queue=w339, element=cluster{"State":string, "Data":variant} {"State"="Search_Drive", "Data"=variant} ("元素")) -> ()  [unwired: 1 in, 4 out]
      }
      event "Read R": Value Change {
        n111 = event-data() -> ()  [unwired: 3 out]
        n112 = Enqueue Element(queue=w341, element=cluster{"State":string, "Data":variant} {"State"="Read_R", "Data"=variant} ("Element")) -> ()  [unwired: 1 in, 4 out]
      }
      event "Creat_Task": Value Change {
        n113 = event-data() -> ()  [unwired: 3 out]
        n114 = Enqueue Element(queue=w343, element=cluster{"State":string, "Data":variant} {"State"="Creat_Task", "Data"=variant} ("Element")) -> ()  [unwired: 1 in, 4 out]
      }
    }
  }
  n115 = Release Queue ("释放队列引用")(queue=w21, force destroy? (F)=TRUE) -> ()  [unwired: 1 in, 3 out]
